vi "zad2.vi"(2 "numer wiersza":i32) -> (0 "sorted array":dbl[](array[numeric]), 1 "Tablica 2d":dbl[][](array[numeric]))   [LabVIEW 2017]
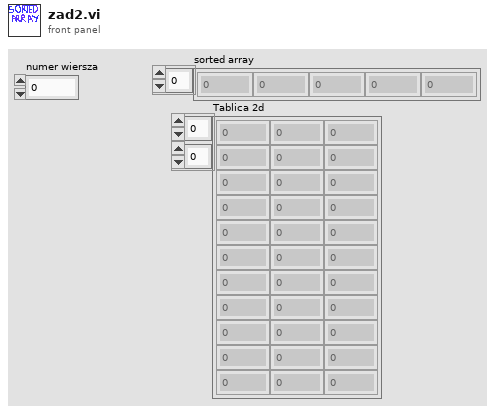
[diagram p1: front panel]
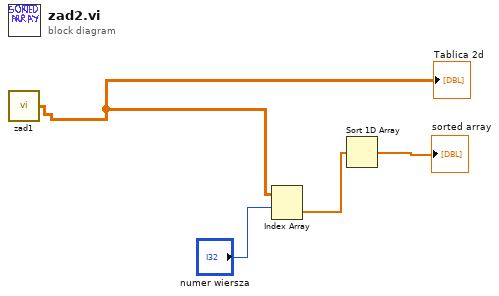
[diagram p0: block diagram]
diagram:
  n1 = call "zad1.vi"() -> ("Tablica 2d"=w2:dbl[][])
  "Tablica 2d" <- w2
  n2 = Index Array(array=w2, index (row)="numer wiersza") -> (element=w4:dbl[])  [unwired: 1 in]
  n3 = Sort 1D Array(array=w4) -> (sorted array=→"sorted array":dbl[])
